vi "TDOA (SubVI).vi"(10 "signal array":dbl[][](array[numeric])) -> (0 "tdoa arrays":dbl[][](array[numeric]), 2 "delay array":dbl[](array[numeric]))   [LabVIEW 2017]
doc: "Vi przyjmuje sygnały z mikrofonów i dla każdej pary oblicza opóźnienie między \"maksimami\", za pomocą Generalized Cross Correlation + Phase Transform (GCC-PHAT). Wynikiem tej operacji jest time delay of arrival (TDOA) każdej z par mikrofonów."
uses:
  <vilib>/Analysis/2dsp.llb/Real FFT.vi
  <vilib>/Analysis/2dsp.llb/Inverse Real FFT.vi
  <vilib>/Analysis/NI_AALPro.lvlib
  <vilib>/Analysis/NI_AAL_SigProc.lvlib
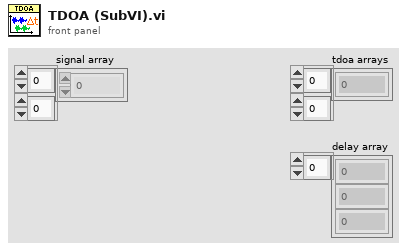
[diagram p1: front panel]
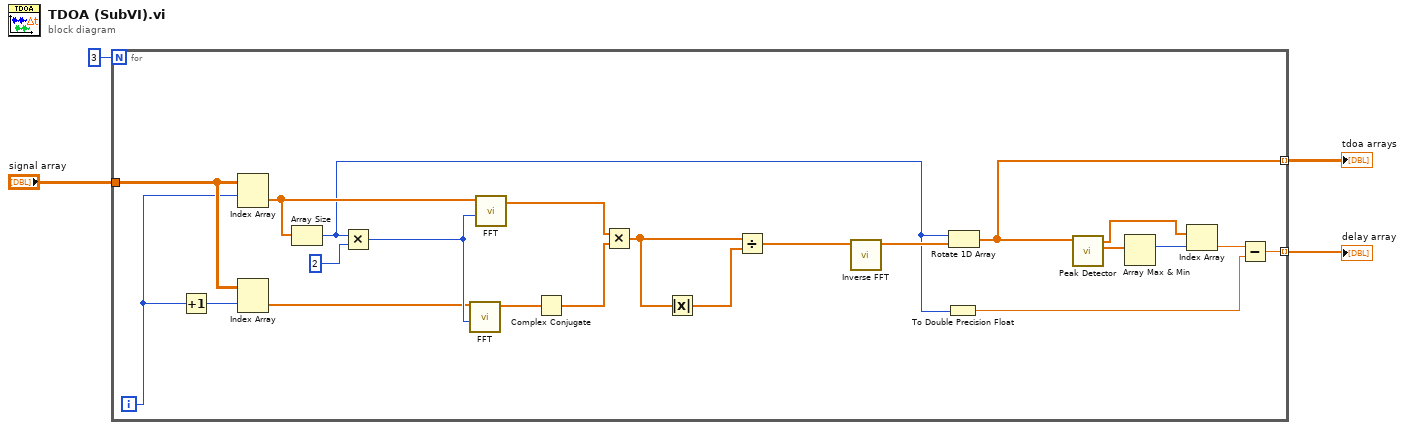
[diagram p0: block diagram]
diagram:
  n1 = for {
    N: 3 -> [_]
    tunnel: "signal array" -> [w26]
    tunnel: [w18] -> w2 mode=indexing
    tunnel: [w16] -> w1 mode=indexing
    i -> [w24]
    n2 = Increment(x=w24) -> (x+1=w25:i32)
    n3 = Index Array(array=w26, index (row)=w24) -> (element=w7:dbl[])  [unwired: 1 in]
    n4 = Index Array(array=w26, index (row)=w25) -> (element=w8:dbl[])  [unwired: 1 in]
    n5 = Array Size(array=w7) -> (size(s)=w6:i32)
    n6 = Multiply(x=w6, y=2) -> (x*y=w15:i32)
    n7 = call-poly <vilib>:"FFT.vi"("FFT size"=w15, "X"=w8) -> ("FFT {X}"=w13:cdb[])  [unwired: 8 in, 1 out]
    n8 = call-poly <vilib>:"FFT.vi"("FFT size"=w15, "X"=w7) -> ("FFT {X}"=w14:cdb[])  [unwired: 8 in, 1 out]
    n9 = Complex Conjugate(1:w13) -> (0:w12:cdb[])
    n10 = Multiply(x=w14, y=w12) -> (x*y=w10:cdb[])
    n11 = Absolute Value(x=w10) -> (abs(x)=w20:dbl[])
    n12 = Divide(x=w10, y=w20) -> (x/y=w9:cdb[])
    n13 = call-poly <vilib>:"Inverse FFT.vi"("FFT {X}"=w9) -> ("X"=w17:dbl[])  [unwired: 9 in, 1 out]
    n14 = To Double Precision Float(number=w6) -> (double precision float=w5:dbl)
    n15 = Rotate 1D Array(1:w17, 2:w6) -> (0:w16:dbl[])
    n16 = call <vilib>:"Peak Detector.vi"("X"=w16) -> ("Amplitudes"=w23:dbl[], "Locations"=w22:dbl[])  [unwired: 6 in, 3 out]
    n17 = Array Max & Min(array=w23) -> (max index (indices)=w21:i32)  [unwired: 3 out]
    n18 = Index Array(array=w22, index=w21) -> (element=w19:dbl)
    n19 = Subtract(x=w19, y=w5) -> (x-y=w18:dbl)
  }
  "delay array" <- w2
  "tdoa arrays" <- w1
